vi "Clear2.vi"(1 "limit 2":T1, 2 "limit":T1, 3 "XYGraphGN":refnum<vi>, 4 "TblRefFormMainShow":refnum<vi>) -> ()   [LabVIEW 2017]
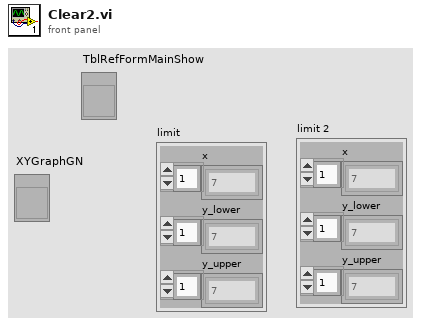
[diagram p1: front panel]
types:
  T1 = cluster{"x":dbl[], "y_lower":dbl[], "y_upper":dbl[]}
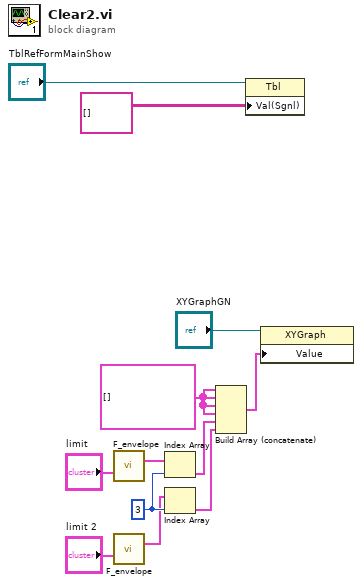
[diagram p0: block diagram]
diagram:
  w4 = 3 ("索引")
  w6 = cluster{dbl[], dbl[]}[] [] ("元素")
  n1 = call "F_envelope.vi"("limit"="limit") -> ("XY_out"=w5:cluster{dbl[], dbl[]}[])  [unwired: 11 in, 3 out]
  n2 = call "F_envelope.vi"("limit"="limit 2") -> ("XY_out"=w3:cluster{dbl[], dbl[]}[])  [unwired: 11 in, 3 out]
  n3 = Index Array(array=w5, index=w4) -> (element=w2:cluster{dbl[], dbl[]})
  n4 = Index Array(array=w3, index=w4) -> (element=w1:cluster{dbl[], dbl[]})
  n5 = Build Array (concatenate)(w6, w6, w6, w6, w2, w1) -> (w8:cluster{dbl[], dbl[]}[])
  n6 = property class="Tbl"(reference="TblRefFormMainShow", "Val(Sgnl)"=string[][] [] ("值(信号)")) -> ()  [unwired: 1 in, 2 out]
  n7 = property class="XYGraph"(reference="XYGraphGN", "Value"=w8) -> ()  [unwired: 1 in, 2 out]
